vi "Attempt Repair.vi"(8 "error in":errorcluster, 11 "CEF_serializable node in":refnum<class "CEF_serializable node.lvclass">) -> (0 "error out":errorcluster, 2 "refresh tree?":bool, 3 "CEF_serializable node out":refnum<class "CEF_serializable node.lvclass">)   [LabVIEW 2023, in "CEF.lvlib" / "CEF_serializable node.lvclass"]
doc: "Copyright 2017 National Instruments Corporation\n\nLicensed under the Apache License, Version 2.0 (the \"License\"); you may not use this file except in compliance with the License. You may obtain a copy of the License at http://www.apache.org/licenses/LICENSE-2.0\nUnless required by applicable law or agreed to in writing, software distributed under the License is distributed on an \"AS IS\" BASIS, WITHOUT WARRANTIES OR CONDITIONS OF ANY KIND, either express or implied. See the License for the specific language governing permissions and limitations under the License."
uses:
  CEF_serializable node.lvclass
  serializable configuration/CEF_serializable configuration.lvclass
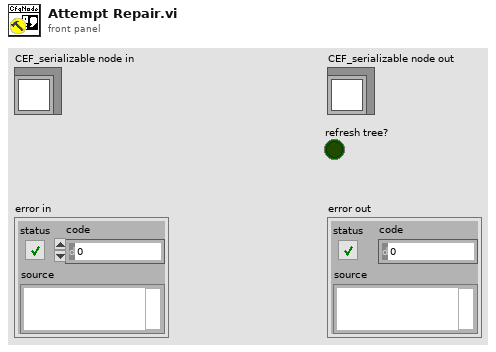
[diagram p1: front panel]
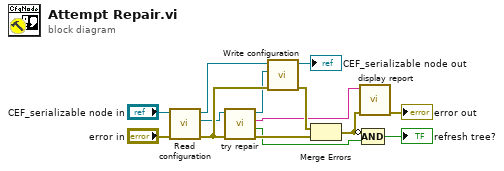
[diagram p0: block diagram]
diagram:
  n1 = call-dynamic "Read configuration.vi"("error in"="error in", "CEF_serializable node in"="CEF_serializable node in") -> ("error out"=w9:errorcluster, "CEF Configuration"=w8:refnum<class "CEF_serializable configuration.lvclass">, "CEF_serializable node out"=w6:refnum<class "CEF_serializable node.lvclass">)  [unwired: 7 in]
  n2 = call "try repair.vi"("error in"=w9, "CEF_Configuration in"=w8) -> ("error out"=w10:errorcluster, "change occurred"=w5:bool, "repair report"=w1:string, "CEF_Configuration out"=w7:refnum<class "CEF_serializable configuration.lvclass">)  [unwired: 6 in]
  n3 = call-dynamic "Write configuration.vi"("error in"=w9, "CEF Configuration"=w7, "CEF_serializable node in"=w6) -> ("error out"=w11:errorcluster, "CEF_serializable node out"=→"CEF_serializable node out":refnum<class "CEF_serializable node.lvclass">)  [unwired: 7 in]
  n4 = Merge Errors(w11, w10) -> (w2:errorcluster)
  n5 = call "display report.vi"("error in"=w2, "data to display"=w1) -> ("error out"=→"error out":errorcluster)  [unwired: 9 in]
  n6 = Compound Arithmetic op=AND(invert w2, w5) -> (→"refresh tree?":bool)
